vi "make_headers.vi"(8 "Error in":errorcluster, 11 "Device In":T1) -> (0 "Error Out":errorcluster, 3 "Device Out":T1)   [LabVIEW 2021]
uses:
  Cluster.ctl
  SHA256/SHA256.lvlib
  <vilib>/Utility/SMTP/NI_SMTPEmail.lvlib
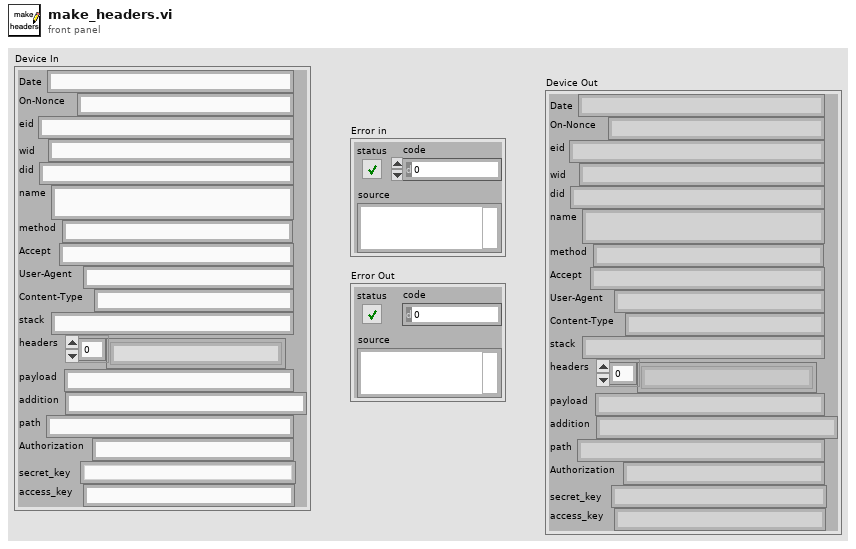
[diagram p1: front panel]
types:
  T1 = typedef "Cluster.ctl" = cluster{"Date":string, "On-Nonce":string, "eid":string, "wid":string, "did":string, "name":string, "method":string, "Accept":string, "User-Agent":string, "Content-Type":string, "stack":string, "headers":string[], "payload":string, "addition":string, "path":string, "Authorization":string, "secret_key":string, "access_key":string}
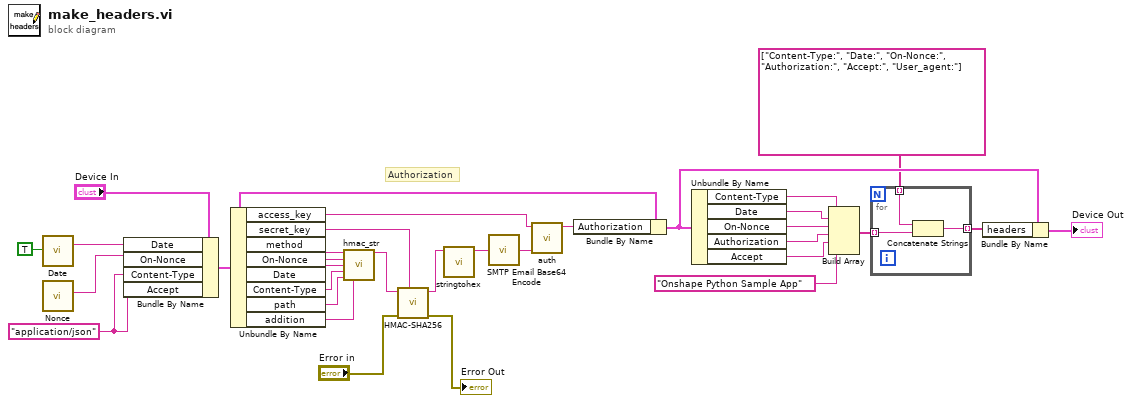
[diagram p0: block diagram]
diagram:
  w10 = "application/json"
  # "Authorization"
  n1 = call "Date.vi"("UTC format"=TRUE) -> ("date/time string"=w21:string)  [unwired: 10 in]
  n2 = call "Nonce.vi"() -> ("Nonce"=w11:string)  [unwired: 11 in]
  n3 = Bundle By Name(cluster="Device In", "Date"=w21, "On-Nonce"=w11, "Content-Type"=w10, "Accept"=w10) -> (w16:T1)
  n4 = Unbundle By Name(w16) -> ("access_key"=w22:string, "secret_key"=w23:string, "method"=w31:string, "On-Nonce"=w30:string, "Date"=w29:string, "Content-Type"=w27:string, "path"=w28:string, "addition"=w12:string)
  n5 = call "hmac_str.vi"("Method"=w31, "Nonce"=w30, "Date"=w29, "ctype"=w27, "path"=w28, "query"=w12) -> ("hmac_str"=w26:string)  [unwired: 9 in]
  n6 = call "HMAC-SHA256.vi"("Key"=w23, "error In"="Error in", "String to Encode"=w26) -> ("error Out"=→"Error Out":errorcluster, "Hash String"=w20:string)  [unwired: 7 in]
  n7 = call "stringtohex.vi"("Hash String"=w20) -> ("string"=w19:string)  [unwired: 10 in]
  n8 = call <vilib>:"SMTP Email Base64 Encode.vi"("Normal String"=w19) -> ("Base64 String"=w25:string)  [unwired: 1 in]
  n9 = call "auth.vi"("signature"=w25, "access_key"=w22) -> ("auth"=w24:string)  [unwired: 9 in]
  n10 = Bundle By Name(cluster=w16, "Authorization"=w24) -> (w15:T1)
  n11 = Unbundle By Name(w15) -> ("Content-Type"=w9:string, "Date"=w8:string, "On-Nonce"=w7:string, "Authorization"=w6:string, "Accept"=w5:string)
  n12 = Build Array(w9, w8, w7, w6, w5, "Onshape Python Sample App" ("string")) -> (w3:string[])
  n13 = for {
    tunnel: string[] ["Content-Type:", "Date:", "On-Nonce:", "Authorization:", "Accept:", "User_agent:"] -> [w35] mode=indexing
    tunnel: w3 -> [w34] mode=indexing
    tunnel: [w33] -> w2 mode=indexing
    n14 = Concatenate Strings(w35, w34) -> (w33:string)
  }
  n15 = Bundle By Name(cluster=w15, "headers"=w2) -> (→"Device Out":T1)
